vi "Get Case Structure Position from VI.vi"(8 "error in (no error)":errorcluster, 11 "Method VI Path":path) -> (0 "error out":errorcluster, 3 "Position":T1)   [LabVIEW 2016, in "SLL Scripting.lvlib" / "SLL Class DVR API Generator.lvlib"]
uses:
  SLL Class DVR API Generator.lvlib
  <vilib>/Utility/miscctls.llb/LVPositionTypeDef.ctl
  <vilib>/Utility/traverseref.llb/TRef TravTarget.ctl
  <vilib>/Utility/traverseref.llb/VI Scripting - Traverse.lvlib
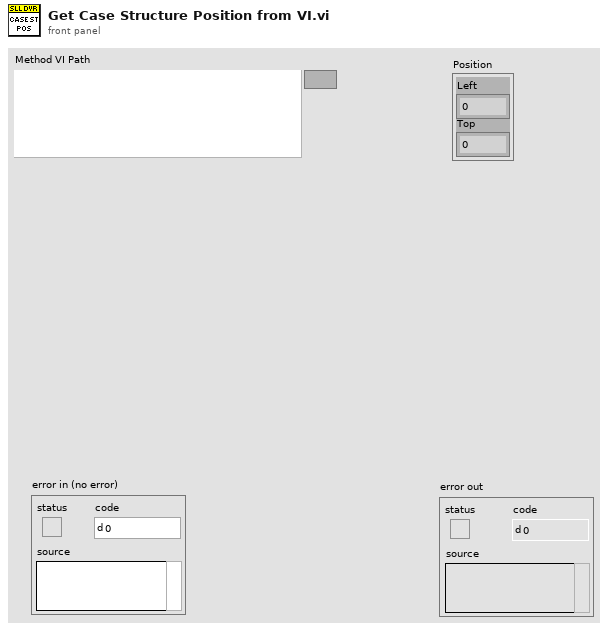
[diagram p1: front panel]
types:
  T1 = typedef "LVPositionTypeDef.ctl" = cluster{"Left":i32, "Top":i32}
  T2 = typedef "TRef TravTarget.ctl" = enum16{"FP", "BD", "Other"}
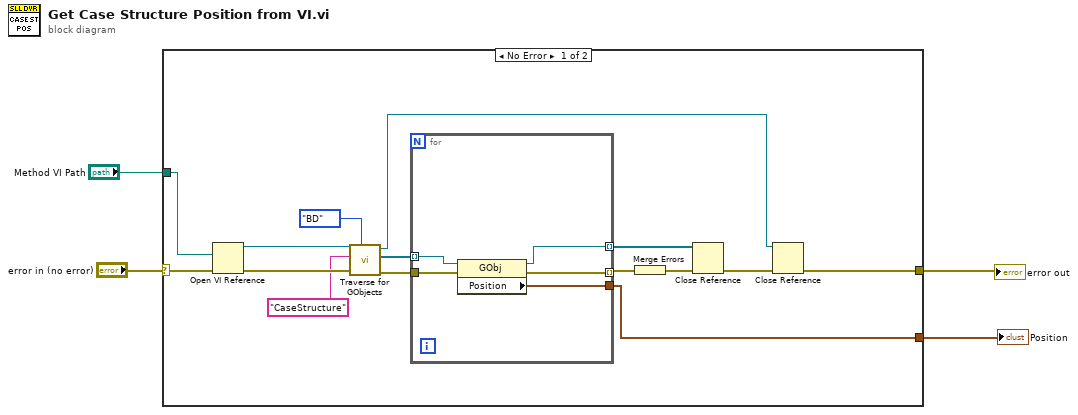
[diagram p0: block diagram]
diagram:
  n1 = case shown="No Error" "error in (no error)" {
    selector: "error in (no error)" -> [w19 w25]
    tunnel: [w6 w25] -> w3
    tunnel: "Method VI Path" -> [w17 _]
    tunnel: [w9 _] -> w1
    frame No Error {
      n2 = Open VI Reference(vi path=w17, error in (no error)=w19) -> (vi reference=w16:refnum<vi>, error out=w18:errorcluster)  [unwired: 4 in]
      n3 = call <vilib>:"Traverse for GObjects.vi"("Traverse Target"=TRef_TravTarget."BD", "error in (no error)"=w18, "Class Name"="CaseStructure", "VI Refnum"=w16) -> ("error out"=w13:errorcluster, "References"=w12:refnum<vi>[], "dup VI Refnum"=w5:refnum<vi>)  [unwired: 4 in, 1 out]
      n4 = for {
        tunnel: w13 -> [w24]
        tunnel: w12 -> [w23] mode=indexing
        tunnel: [w22] -> w11 mode=indexing
        tunnel: [w21] -> w9
        tunnel: [w20] -> w7 mode=indexing
        n5 = property class="GObj"(reference=w23, error in=w24) -> (reference out=w20:refnum<vi>, error out=w22:errorcluster, "Position"=w21:T1)
      }
      n6 = Merge Errors(w11) -> (w10:errorcluster)
      n7 = Close Reference(reference=w7, error in (no error)=w10) -> (error out=w8:errorcluster)
      n8 = Close Reference(reference=w5, error in (no error)=w8) -> (error out=w6:errorcluster)
    }
    frame Error {
    }
  }
  "error out" <- w3
  "Position" <- w1
